vi "Notifier_Driver.vi"(0 "Notification":bool, 2 "Name":string, 11 "Error_In":errorcluster, 13 "Notifier_Operation_Select":T1=enum."Send_Notification") -> (4 "Latest_Notification":bool, 15 "Error_Out":errorcluster)   [LabVIEW 2023]
uses:
  Controls/Notifier_Operation_Select.ctl
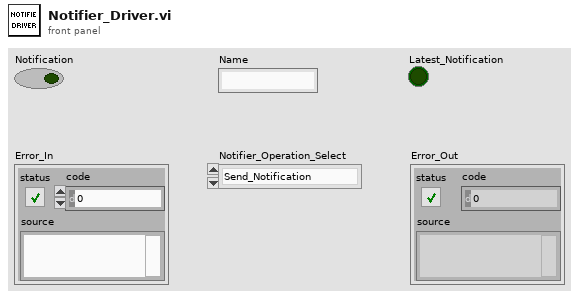
[diagram p1: front panel]
types:
  T1 = typedef "Notifier_Operation_Select.ctl" = enum16{"Obtain_Notifier", "Send_Notification", "Get_Notification_Status", "Release_Notifier"}
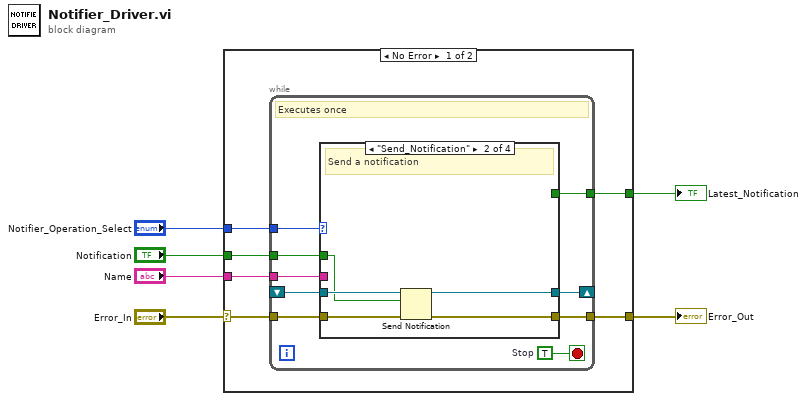
[diagram p0: block diagram]
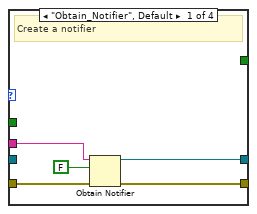
[diagram p2: hidden frame]
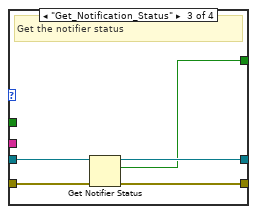
[diagram p3: hidden frame]
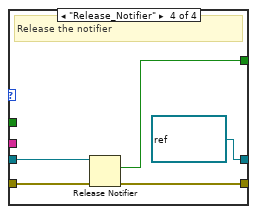
[diagram p4: hidden frame]
diagram:
  n1 = case shown="No Error" "Error_In" {
    selector: "Error_In" -> [w12 w42]
    tunnel: [w11 w42] -> w5
    tunnel: "Notifier_Operation_Select" -> [w10 _]
    tunnel: "Name" -> [w9 _]
    tunnel: "Notification" -> [w8 _]
    tunnel: [w7 _] -> w1
    frame No Error {
      n2 = while {
        tunnel: w12 -> [w21]
        tunnel: [w20] -> w11
        tunnel: w10 -> [w19]
        tunnel: w9 -> [w18]
        shift-right: [w17] -> _
        shift-left: _ -> [w16]
        tunnel: w8 -> [w15]
        tunnel: [w14] -> w7
        stop <- w13 stop-if-true
        w13 = TRUE  # Stop
        # "Executes once"
        n3 = case shown="\"Send_Notification\"" w19 {
          tunnel: w21 -> [w26 w31 w36 w41]
          tunnel: [w25 w30 w35 w40] -> w20
          tunnel: w18 -> [w24 _ _ _]
          tunnel: [w22 w28 w33 refnum<notifier> refnum ("notifier out")] -> w17
          tunnel: w16 -> [_ w29 w34 w39]
          tunnel: w15 -> [_ w27 _ _]
          tunnel: [_ _ w32 w38] -> w14
          frame "Obtain_Notifier", Default {
            # "Create a notifier"
            n4 = Obtain Notifier(name (unnamed)=w24, notification data type=FALSE, error in (no error)=w26) -> (notifier out=w22:refnum<notifier>, error out=w25:errorcluster)  [unwired: 1 in, 1 out]
          }
          frame "Send_Notification" {
            # "Send a notification"
            n5 = Send Notification(notification=w27, notifier=w29, error in (no error)=w31) -> (notifier out=w28:refnum<notifier>, error out=w30:errorcluster)
          }
          frame "Get_Notification_Status" {
            # "Get the notifier status"
            n6 = Get Notifier Status(notifier=w34, error in (no error)=w36) -> (notifier out=w33:refnum<notifier>, current notification=w32:bool, error out=w35:errorcluster)  [unwired: 2 out]
          }
          frame "Release_Notifier" {
            # "Release the notifier"
            n7 = Release Notifier(notifier=w39, error in (no error)=w41) -> (last notification=w38:bool, error out=w40:errorcluster)  [unwired: 1 in, 1 out]
          }
        }
      }
    }
    frame Error {
    }
  }
  "Error_Out" <- w5
  "Latest_Notification" <- w1
